vi "Maths - Cpk.vi"(7 "Plots (True)":bool=TRUE, 9 "Results":dbl[](array[numeric])=[4.0, 4.1, 4.07, 4.1, 4.0, 4.05, 4.3, 3.97], 10 "Upper Limit":dbl=5.0, 11 "Lower Limit":dbl=3.0) -> (2 "Results":T1={"Target"=4.0, "Average"=4.07375, "Standard Deviation"=0.10336309095334055, "Cp"=3.2248777610937, "Cpu"=2.9870430262130383, "Cpl"=3.462712495974362, "Cpk"=2.9870430262130383}, 4 "Graph":picture, 6 "Histogram":picture)   [LabVIEW 2010]
uses:
  <vilib>/Analysis/NI_AALBase.lvlib
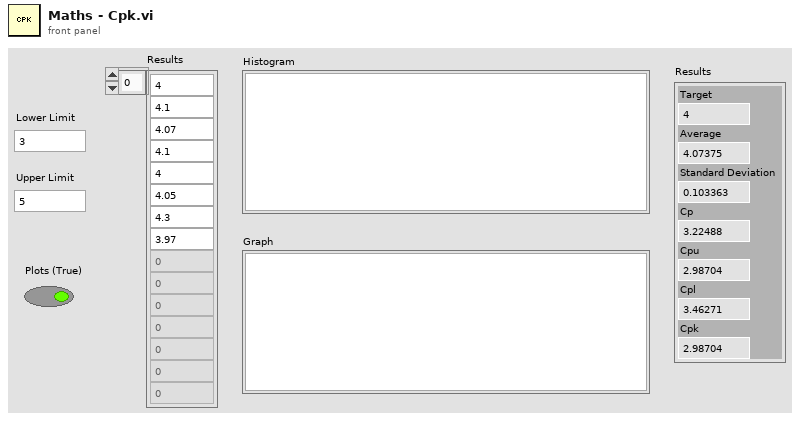
[diagram p1: front panel]
types:
  T1 = cluster{"Target":dbl, "Average":dbl, "Standard Deviation":dbl, "Cp":dbl, "Cpu":dbl, "Cpl":dbl, "Cpk":dbl}
  T2 = cluster{"left":i16, "top":i16, "right":i16, "bottom":i16}
  T3 = cluster{"horizontal":enum16{"left", "center", "right"}, "vertical":enum16{"top", "center", "bottom"}}
  T4 = cluster{"Width":i16, "Style":enum32{"Solid", "Dash", "Dot", "DashDot", "DashDotDot"}}
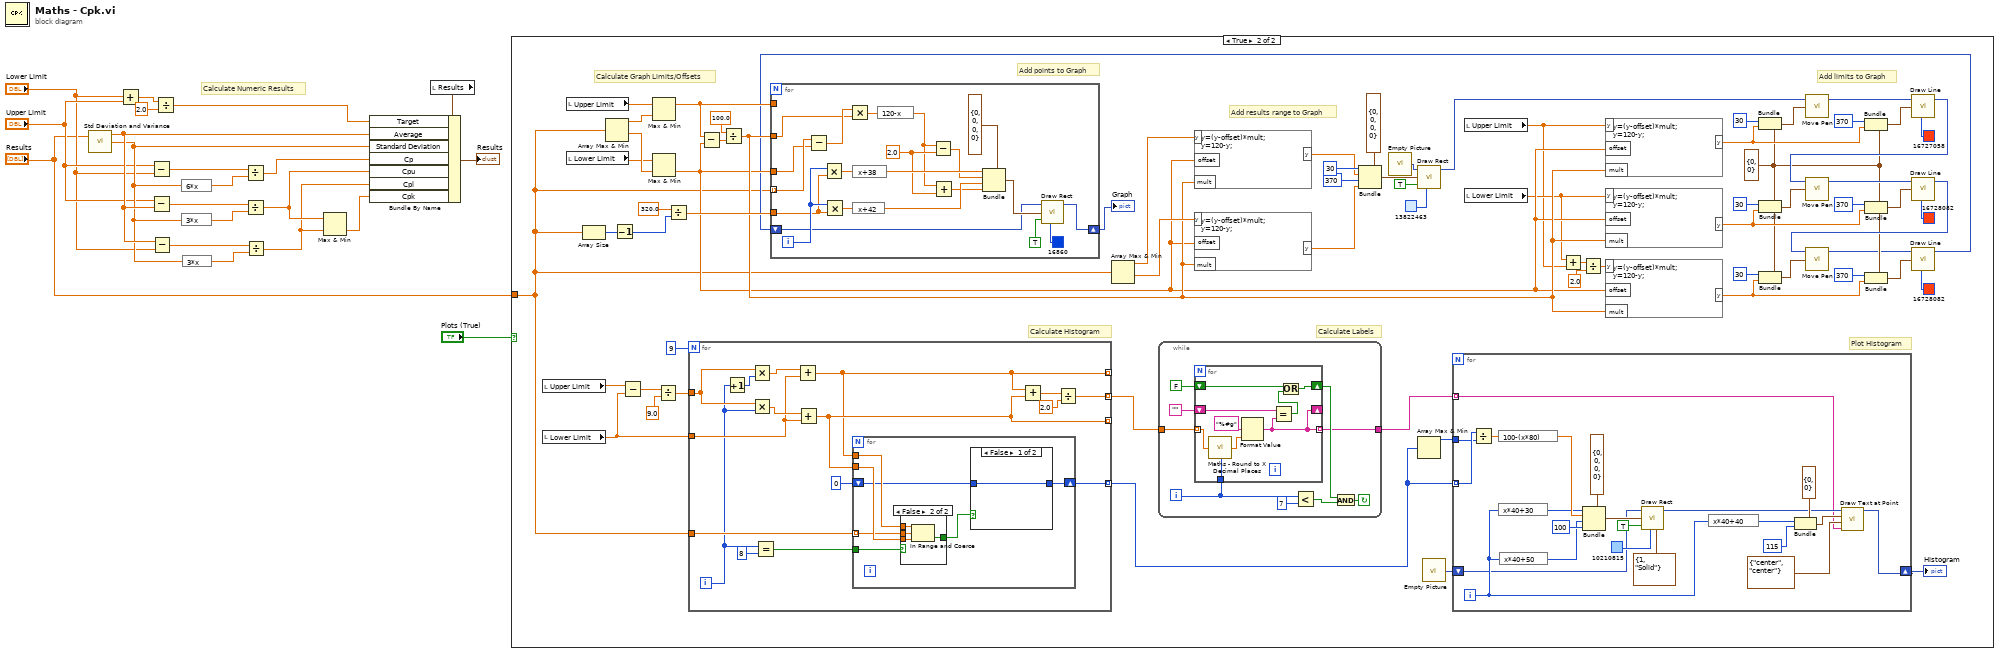
[diagram p0: block diagram]
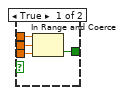
[diagram p3: hidden frame]
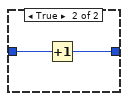
[diagram p4: hidden frame]
diagram:
  # "Calculate Numeric Results"
  n1 = call <vilib>:"Std Deviation and Variance.vi"("X"="Results") -> ("mean"=w10:dbl, "standard deviation"=w9:dbl)  [unwired: 1 in, 1 out]
  n2 = Add(x="Lower Limit", y="Upper Limit") -> (x+y=w21:dbl)
  n3 = Subtract(x="Upper Limit", y="Lower Limit") -> (x-y=w19:dbl)
  n4 = Subtract(x="Upper Limit", y=w10) -> (x-y=w16:dbl)
  n5 = Subtract(x=w10, y="Lower Limit") -> (x-y=w15:dbl)
  n6 = Divide(x=w21, y=2.0) -> (x/y=w11:dbl)
  n7 = expression code="6*x"(w9) -> (w18:dbl)
  n8 = expression code="3*x"(w9) -> (w17:dbl)
  n9 = expression code="3*x"(w9) -> (w14:dbl)
  n10 = Divide(x=w19, y=w18) -> (x/y=w8:dbl)
  n11 = Divide(x=w16, y=w17) -> (x/y=w7:dbl)
  n12 = Divide(x=w15, y=w14) -> (x/y=w6:dbl)
  n13 = Max & Min(x=w7, y=w6) -> (min(x,y)=w5:dbl)  [unwired: 1 out]
  n14 = local read "Results"() -> (w12:T1)
  n15 = Bundle By Name(cluster=w12, "Target"=w11, "Average"=w10, "Standard Deviation"=w9, "Cp"=w8, "Cpu"=w7, "Cpl"=w6, "Cpk"=w5) -> (→"Results":T1)
  n16 = case shown="True" "Plots (True)" {
    tunnel: "Results" -> [_ w27]
    frame False {
    }
    frame True {
      w29 = cluster{"x":i16, "y":i16} {"x"=0, "y"=0} ("new position")
      # "Calculate Labels"
      # "Add results range to Graph"
      # "Add limits to Graph"
      # "Calculate Graph Limits/Offsets"
      # "Add points to Graph"
      # "Plot Histogram"
      # "Calculate Histogram"
      n17 = local read "Upper Limit"() -> (w26:dbl)
      n18 = local read "Lower Limit"() -> (w25:dbl)
      n19 = local read "Upper Limit"() -> (w83:dbl)
      n20 = local read "Lower Limit"() -> (w80:dbl)
      n21 = Array Size(array=w27) -> (size(s)=w77:i32)
      n22 = Array Max & Min(array=w27) -> (max value=w82:dbl, min value=w81:dbl)  [unwired: 2 out]
      n23 = Decrement(x=w77) -> (x-1=w62:i32)
      n24 = Subtract(x=w26, y=w25) -> (x-y=w90:dbl)
      n25 = Max & Min(x=w83, y=w82) -> (max(x,y)=w79:dbl)  [unwired: 1 out]
      n26 = Max & Min(x=w80, y=w81) -> (min(x,y)=w37:dbl)  [unwired: 1 out]
      n27 = Divide(x=w90, y=9.0) -> (x/y=w87:dbl)
      n28 = Divide(x=320.0, y=w62) -> (x/y=w75:dbl)
      n29 = for {
        N: 9 -> [_]
        tunnel: w87 -> [w166]
        tunnel: w25 -> [w157]
        tunnel: [w160] -> _ mode=indexing
        tunnel: [w158] -> _ mode=indexing
        tunnel: [w153] -> w24 mode=indexing
        tunnel: w27 -> [w162]
        tunnel: [w152] -> w22 mode=indexing
        i -> [w154]
        n30 = Increment(x=w154) -> (x+1=w165:i32)
        n31 = Multiply(x=w166, y=w165) -> (x*y=w159:dbl)
        n32 = Multiply(x=w166, y=w154) -> (x*y=w167:dbl)
        n33 = Equal?(x=w154, y=8) -> (x = y?=w155:bool)
        n34 = Add(x=w159, y=w157) -> (x+y=w158:dbl)
        n35 = Add(x=w167, y=w157) -> (x+y=w160:dbl)
        n36 = for {
          tunnel: w162 -> [w172] mode=indexing
          shift-right: [w169] -> w152
          shift-left: 0 -> [w170]
          tunnel: w160 -> [w174]
          tunnel: w158 -> [w173]
          tunnel: w155 -> [w168]
          n37 = case shown="False" w168 {
            tunnel: w174 -> [w178 w182]
            tunnel: w173 -> [w177 w181]
            tunnel: w172 -> [w176 w180]
            tunnel: [w175 w179] -> w171
            frame True {
              n38 = In Range and Coerce(upper limit=w177, x=w176, lower limit=w178) -> (In Range?=w175:bool)  [unwired: 1 out]
            }
            frame False {
              n39 = In Range and Coerce(upper limit=w181, x=w180, lower limit=w182) -> (In Range?=w179:bool)  [unwired: 1 out]
            }
          }
          n40 = case shown="False" w171 {
            tunnel: w170 -> [w183 w185]
            tunnel: [w183 w184] -> w169
            frame False {
            }
            frame True {
              n41 = Increment(x=w185) -> (x+1=w184:i32)
            }
          }
        }
        n42 = Add(x=w158, y=w160) -> (x+y=w164:dbl)
        n43 = Divide(x=w164, y=2.0) -> (x/y=w153:dbl)
      }
      n44 = Subtract(x=w79, y=w37) -> (x-y=w78:dbl)
      n45 = Divide(x=100.0, y=w78) -> (x/y=w38:dbl)
      n46 = Array Max & Min(array=w27) -> (max value=w48:dbl, min value=w49:dbl)  [unwired: 2 out]
      n47 = while {
        tunnel: w24 -> [w99]
        tunnel: [w92] -> w23
        i -> [w91]
        stop <- w96 continue-if-true
        n48 = for {
          tunnel: w99 -> [w103] mode=indexing
          tunnel: [w104] -> w92 mode=indexing
          shift-right: [w104] -> _
          shift-left: "" -> [w108]
          shift-right: [w106] -> w95
          shift-left: FALSE -> [w107]
          tunnel: w91 -> [w100]
          n49 = call "Maths - Round to X Decimal Places.vi"("Floating In"=w103, "Decimal Places (2)"=w100) -> ("Floating Out"=w101:dbl)
          n50 = Format Value(format string="%#g", value (0)=w101) -> (output string=w104:string)  [unwired: 1 in]
          n51 = Equal?(x=w108, y=w104) -> (x = y?=w105:bool)
          n52 = Or(x=w107, y=w105) -> (x .or. y?=w106:bool)
        }
        n53 = Less?(x=w91, y=7) -> (x < y?=w93:bool)
        n54 = And(x=w95, y=w93) -> (x .and. y?=w96:bool)
      }
      n55 = formula code="y=(y-offset)*mult;\ny=120-y;"("y"=w48, "offset"=w37, "mult"=w38) -> ("y"=w52:dbl)
      n56 = formula code="y=(y-offset)*mult;\ny=120-y;"("y"=w49, "offset"=w37, "mult"=w38) -> ("y"=w51:dbl)
      n57 = Bundle(cluster=T2 {"left"=0, "top"=0, "right"=0, "bottom"=0} ("rect"), "left"=i16 30, "top"=w52, "right"=i16 370, "bottom"=w51) -> (w57:T2)
      n58 = call "Empty Picture"() -> ("empty picture"=w47:picture)
      n59 = call <vilib>:"Draw Rect.vi"("picture"=w47, "rect"=w57, "fill?(F)"=TRUE, "color(black)"=u32 13822463) -> ("new picture"=w45:picture)  [unwired: 5 in]
      n60 = Array Max & Min(array=w22) -> (max value=w84:i32)  [unwired: 3 out]
      n61 = call "Empty Picture"() -> ("empty picture"=w86:picture)
      n62 = for {
        shift-right: [w135] -> w85
        shift-left: w86 -> [w134]
        tunnel: w23 -> [w130] mode=indexing
        tunnel: w22 -> [w133] mode=indexing
        tunnel: w84 -> [w132]
        i -> [w136]
        n63 = Divide(x=w133, y=w132) -> (x/y=w131:dbl)
        n64 = expression code="100-(x*80)"(w131) -> (w141:dbl)
        n65 = expression code="x*40+30"(w136) -> (w139:i32)
        n66 = expression code="x*40+50"(w136) -> (w140:i32)
        n67 = Bundle(cluster=T2 {"left"=0, "top"=0, "right"=0, "bottom"=0} ("rect"), "left"=w139, "top"=w141, "right"=w140, "bottom"=i16 100) -> (w137:T2)
        n68 = call <vilib>:"Draw Rect.vi"("picture"=w134, "rect"=w137, "fill?(F)"=TRUE, "color(black)"=u32 10210815, "pen"=T4 {"Width"=1, "Style"=enum."Solid"}) -> ("new picture"=w146:picture)  [unwired: 4 in]
        n69 = expression code="x*40+40"(w136) -> (w149:i32)
        n70 = Bundle(cluster=cluster{"x":i16, "y":i16} {"x"=0, "y"=0} ("origin"), "x"=w149, "y"=i16 115) -> (w148:cluster{"x":i16, "y":i16})
        n71 = call <vilib>:"Draw Text at Point.vi"("text"=w130, "alignment(left, top)"=T3 {"horizontal"=enum."center", "vertical"=enum."center"}, "origin"=w148, "picture"=w146) -> ("new picture"=w135:picture)  [unwired: 6 in, 1 out]
      }
      "Histogram" <- w85
      n72 = local read "Upper Limit"() -> (w32:dbl)
      n73 = local read "Lower Limit"() -> (w33:dbl)
      n74 = Add(x=w33, y=w32) -> (x+y=w36:dbl)
      n75 = Divide(x=w36, y=2.0) -> (x/y=w34:dbl)
      n76 = formula code="y=(y-offset)*mult;\ny=120-y;"("y"=w32, "offset"=w37, "mult"=w38) -> ("y"=w59:dbl)
      n77 = formula code="y=(y-offset)*mult;\ny=120-y;"("y"=w33, "offset"=w37, "mult"=w38) -> ("y"=w58:dbl)
      n78 = formula code="y=(y-offset)*mult;\ny=120-y;"("y"=w34, "offset"=w37, "mult"=w38) -> ("y"=w44:dbl)
      n79 = Bundle(cluster=w29, "x"=i16 30, "y"=w59) -> (w70:cluster{"x":i16, "y":i16})
      n80 = Bundle(cluster=w29, "x"=i16 30, "y"=w58) -> (w68:cluster{"x":i16, "y":i16})
      n81 = Bundle(cluster=w29, "x"=i16 30, "y"=w44) -> (w39:cluster{"x":i16, "y":i16})
      n82 = call <vilib>:"Move Pen.vi"("new position"=w70, "picture"=w45) -> ("new picture"=w73:picture)  [unwired: 3 in]
      n83 = Bundle(cluster=w29, "x"=i16 370, "y"=w59) -> (w66:cluster{"x":i16, "y":i16})
      n84 = Bundle(cluster=w29, "x"=i16 370, "y"=w58) -> (w65:cluster{"x":i16, "y":i16})
      n85 = Bundle(cluster=w29, "x"=i16 370, "y"=w44) -> (w41:cluster{"x":i16, "y":i16})
      n86 = call <vilib>:"Draw Line.vi"("picture"=w73, "end point"=w66, "color(black)"=u32 16727058) -> ("new picture"=w72:picture)  [unwired: 6 in]
      n87 = call <vilib>:"Move Pen.vi"("new position"=w68, "picture"=w72) -> ("new picture"=w71:picture)  [unwired: 3 in]
      n88 = call <vilib>:"Draw Line.vi"("picture"=w71, "end point"=w65, "color(black)"=u32 16728082) -> ("new picture"=w30:picture)  [unwired: 6 in]
      n89 = call <vilib>:"Move Pen.vi"("new position"=w39, "picture"=w30) -> ("new picture"=w28:picture)  [unwired: 3 in]
      n90 = call <vilib>:"Draw Line.vi"("picture"=w28, "end point"=w41, "color(black)"=u32 16728082) -> ("new picture"=w31:picture)  [unwired: 6 in]
      n91 = for {
        shift-right: [w124] -> w46
        shift-left: w31 -> [w123]
        tunnel: w79 -> [_]
        tunnel: w37 -> [w120]
        tunnel: w27 -> [w121] mode=indexing
        tunnel: w38 -> [w116]
        tunnel: w75 -> [w112]
        i -> [w126]
        w118 = 2.0 ("y")
        n92 = Subtract(x=w121, y=w120) -> (x-y=w122:dbl)
        n93 = Multiply(x=w126, y=w112) -> (x*y=w113:dbl)
        n94 = Multiply(x=w126, y=w112) -> (x*y=w111:dbl)
        n95 = Multiply(x=w122, y=w116) -> (x*y=w115:dbl)
        n96 = expression code="x+38"(w113) -> (w127:dbl)
        n97 = expression code="x+42"(w111) -> (w125:dbl)
        n98 = expression code="120-x"(w115) -> (w114:dbl)
        n99 = Subtract(x=w114, y=w118) -> (x-y=w119:dbl)
        n100 = Add(x=w114, y=w118) -> (x+y=w117:dbl)
        n101 = Bundle(cluster=T2 {"left"=0, "top"=0, "right"=0, "bottom"=0} ("rect"), "left"=w127, "top"=w119, "right"=w125, "bottom"=w117) -> (w129:T2)
        n102 = call <vilib>:"Draw Rect.vi"("picture"=w123, "rect"=w129, "fill?(F)"=TRUE, "color(black)"=u32 16860) -> ("new picture"=w124:picture)  [unwired: 5 in]
      }
      "Graph" <- w46
    }
  }
